vi "LWXPS_GatheringExternalConfigurationSet.vi"(0 "XPS Reference IN":refnum<k24>, 5 "Gathering Type IN":string[](array[string]), 11 "LabVIEW error IN":errorcluster) -> (4 "XPS Reference OUT":refnum<k24>, 6 "Returned error code":i32, 8 "Gathering Type OUT":string[](array[string]), 10 "XPS Error String":string, 15 "LabVIEW error OUT":errorcluster)   [LabVIEW 2014]
uses:
  D:/XPSQ8_LabView_Library/Development/Source/Dll/Newport.XPS.CommandInterface.dll
  Dll/Newport.XPS.CommandInterface.dll
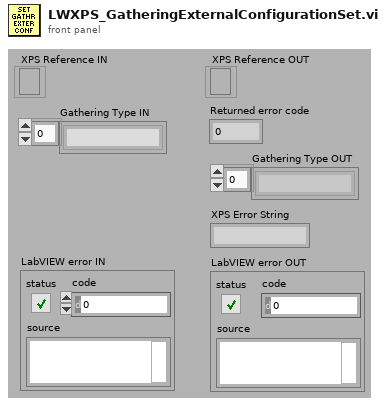
[diagram p1: front panel]
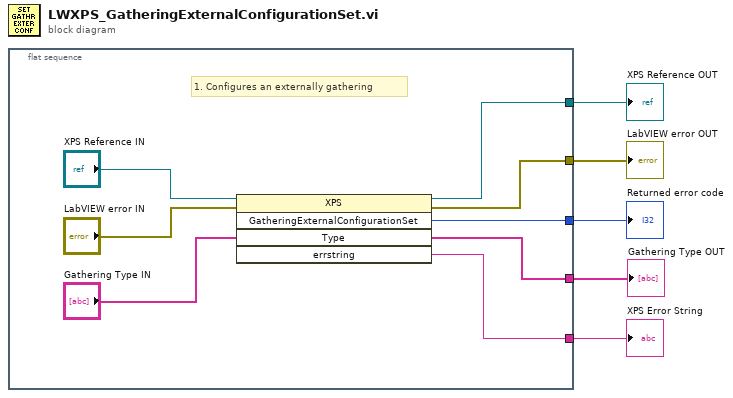
[diagram p0: block diagram]
diagram:
  n1 = flat-sequence {
    tunnel: [w12] -> w5
    tunnel: [w11] -> w4
    tunnel: [w10] -> w3
    tunnel: [w7] -> w2
    tunnel: [w8] -> w1
    frame #0 {
      # "1. Configures an externally gathering"
      n2 = invoke class="XPS" method="GatheringExternalConfigurationSet"(reference="XPS Reference IN", error in="LabVIEW error IN", "Type"="Gathering Type IN") -> (reference out=w12:refnum<k24>, error out=w11:errorcluster, "GatheringExternalConfigurationSet"=w10:i32, "Type"=w8:string[], "errstring"=w7:string)  [unwired: 2 in]
    }
  }
  "XPS Reference OUT" <- w5
  "LabVIEW error OUT" <- w4
  "Returned error code" <- w3
  "XPS Error String" <- w2
  "Gathering Type OUT" <- w1
